vi "VPA QC Config IO.vi"(0 "XDCR 1 Offset":dbl, 1 "Function":enum16{"Read", "Write"}(ring), 5 "XDCR 1 Scale":dbl, 7 "XDCR 2 Offset":dbl, 9 "XDCR 2 Scale":dbl) -> (3 "refnum out":T1, 4 "XDCR 1 Offset":dbl, 6 "XDCR 1 Scale":dbl, 8 "XDCR 2 Offset":dbl, 10 "XDCR 2 Scale":dbl)   [LabVIEW 2013]
uses:
  <vilib>/Utility/config.llb/Config Data RefNum.ctl
  <vilib>/Utility/sysdir.llb/System Directory Type.ctl
  <vilib>/Utility/config.llb/Read Key (Double).vi
  <vilib>/Utility/config.llb/Write Key (Double).vi
  <vilib>/Utility/config.llb/NI_LVConfig.lvlib
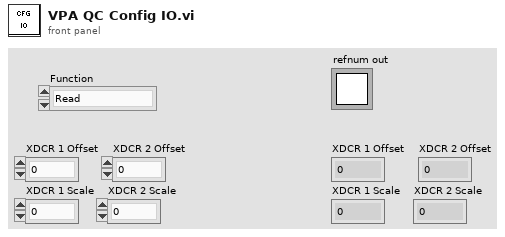
[diagram p1: front panel]
types:
  T1 = typedef "NI_LVConfig.lvlib/Config Data RefNum.ctl" = refnum<k1>
  T2 = typedef "System Directory Type.ctl" = i32
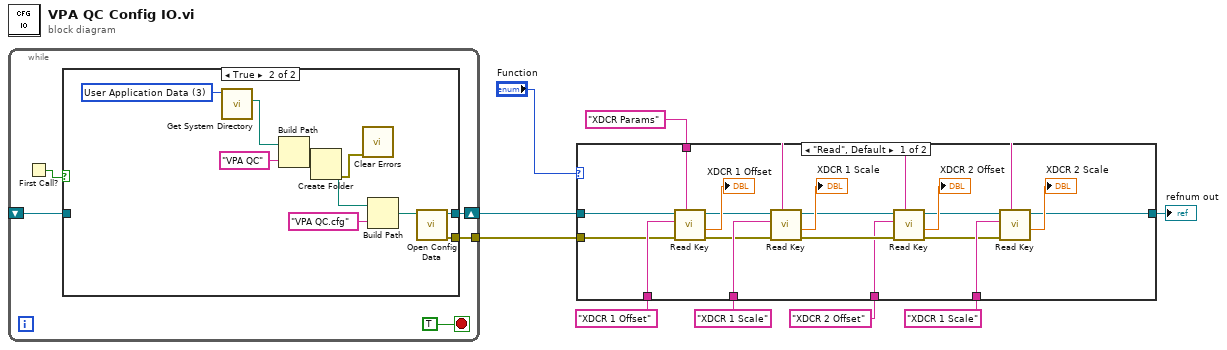
[diagram p0: block diagram]
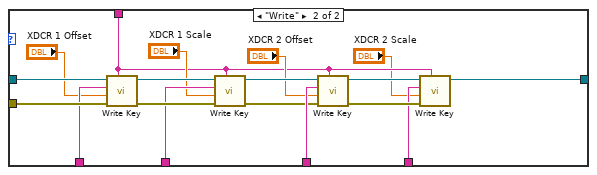
[diagram p2: hidden frame]
diagram:
  n1 = while {
    tunnel: [w13] -> w3
    shift-right: [w14] -> w9
    shift-left: _ -> [w10]
    stop <- TRUE stop-if-true
    n2 = First Call?() -> (First Call?: T/F=w11:bool)
    n3 = case shown="True" w11 {
      tunnel: [w15 w17] -> w14
      tunnel: [_ w16] -> w13
      tunnel: w10 -> [w15 _]
      frame False {
      }
      frame True {
        w18 = T2 3 items=["User Home"=0, "User Desktop"=1, "User Documents"=2, "User Application Data"=3, "User Preferences"=4, "User Temporary"=5, "Public Documents"=6, "Public Application Data"=7, "Public Preferences"=8, "Public Cache"=13, "System Core Libraries"=9, "System Installed Libraries"=10, "Application Files"=11, "Boot Volume Root"=12] ("system directory type")
        n4 = call <vilib>:"Get System Directory.vi"("system directory type"=w18) -> ("system directory"=w19:path)  [unwired: 10 in]
        n5 = Build Path(base path=w19, name or relative path="VPA QC") -> (appended path=w21:path)
        n6 = Create Folder(path (use dialog)=w21) -> (created path=w23:path, error out=w22:errorcluster)  [unwired: 2 in, 1 out]
        n7 = call <vilib>:"Clear Errors.vi"("error in (no error)"=w22) -> ()  [unwired: 6 in, 1 out]
        n8 = Build Path(base path=w23, name or relative path="VPA QC.cfg") -> (appended path=w25:path)
        n9 = call <vilib>:"Open Config Data.vi"("configuration file path"=w25) -> ("error out"=w16:errorcluster, "refnum"=w17:T1)  [unwired: 8 in, 1 out]
      }
    }
  }
  n10 = case shown="\"Read\", Default" "Function" {
    tunnel: w9 -> [w43 w61]
    tunnel: "XDCR 1 Offset" ("key") -> [w42 w59]
    tunnel: "XDCR 1 Scale" ("key") -> [w39 w55]
    tunnel: "XDCR 2 Offset" ("key") -> [w34 w53]
    tunnel: "XDCR Params" ("section") -> [w31 w46]
    tunnel: "XDCR 1 Scale" ("key") -> [w30 w47]
    tunnel: w3 -> [w28 w60]
    tunnel: [w26 w44] -> w1
    frame "Read", Default {
      n11 = call-poly <vilib>:"Read Key.vi"("section"=w31, "error in (no error)"=w28, "key"=w42, "refnum"=w43) -> ("error out"=w36:errorcluster, "value"=→"XDCR 1 Offset":dbl, "refnum out"=w40:T1)  [unwired: 4 in, 1 out]
      n12 = call-poly <vilib>:"Read Key.vi"("section"=w31, "error in (no error)"=w36, "key"=w39, "refnum"=w40) -> ("error out"=w35:errorcluster, "value"=→"XDCR 1 Scale":dbl, "refnum out"=w37:T1)  [unwired: 4 in, 1 out]
      n13 = call-poly <vilib>:"Read Key.vi"("section"=w31, "error in (no error)"=w35, "key"=w34, "refnum"=w37) -> ("error out"=w29:errorcluster, "value"=→"XDCR 2 Offset":dbl, "refnum out"=w32:T1)  [unwired: 4 in, 1 out]
      n14 = call-poly <vilib>:"Read Key.vi"("section"=w31, "error in (no error)"=w29, "key"=w30, "refnum"=w32) -> ("value"=→"XDCR 2 Scale":dbl, "refnum out"=w26:T1)  [unwired: 4 in, 2 out]
    }
    frame "Write" {
      n15 = call-poly <vilib>:"Write Key.vi"("section"=w46, "error in (no error)"=w60, "value"="XDCR 1 Offset", "key"=w59, "refnum"=w61) -> ("error out"=w56:errorcluster, "refnum out"=w57:T1)  [unwired: 4 in, 1 out]
      n16 = call-poly <vilib>:"Write Key.vi"("section"=w46, "error in (no error)"=w56, "value"="XDCR 1 Scale", "key"=w55, "refnum"=w57) -> ("error out"=w51:errorcluster, "refnum out"=w52:T1)  [unwired: 4 in, 1 out]
      n17 = call-poly <vilib>:"Write Key.vi"("section"=w46, "error in (no error)"=w51, "value"="XDCR 2 Offset", "key"=w53, "refnum"=w52) -> ("error out"=w48:errorcluster, "refnum out"=w49:T1)  [unwired: 4 in, 1 out]
      n18 = call-poly <vilib>:"Write Key.vi"("section"=w46, "error in (no error)"=w48, "value"="XDCR 2 Scale", "key"=w47, "refnum"=w49) -> ("refnum out"=w44:T1)  [unwired: 4 in, 2 out]
    }
  }
  "refnum out" <- w1
